vi "Mediaplayer Stop.vi"(2 "MediaPlayer":refnum<k7>(container), 3 "error in":errorcluster) -> (7 "error out":errorcluster)   [LabVIEW 2010]
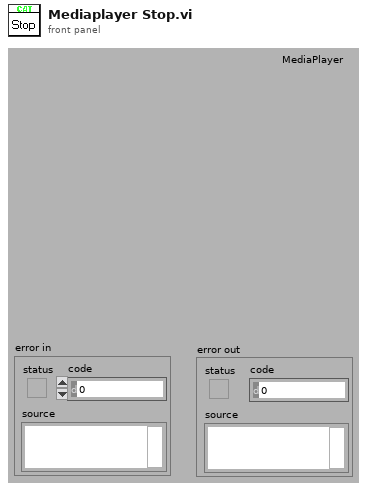
[diagram p1: front panel]
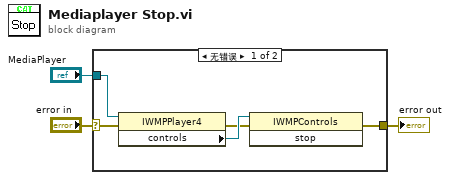
[diagram p0: block diagram]
diagram:
  n1 = case shown="无错误" "error in" {
    selector: "error in" -> [w4 w9]
    tunnel: [w7 w9] -> w3
    tunnel: "MediaPlayer" -> [w8 _]
    frame No Error {
      n2 = property class="IWMPPlayer4"(reference=w8, error in=w4) -> (error out=w5:errorcluster, "controls"=w6:refnum<k7>)  [unwired: 1 out]
      n3 = invoke class="IWMPControls" method="stop"(reference=w6, error in=w5) -> (error out=w7:errorcluster)  [unwired: 1 in, 2 out]
    }
    frame Error {
    }
  }
  "error out" <- w3
